vi "Bridge Null Offset.vi"(8 "error in (no error)":errorcluster, 11 "DAQmxAI in":refnum<class "DAQmxAI.lvclass">) -> (0 "error out":errorcluster, 3 "DAQmxAI out":refnum<class "DAQmxAI.lvclass">)   [LabVIEW 2023, in "VolatusDAQ.lvlib" / "DAQmxAI.lvclass"]
uses:
  DAQmxAI.lvclass
  DAQmxAI.lvclass/DAQmxAI.ctl
  Volatus/Module/Module.lvclass
  lv-vecto/Vecto/Group DBL/Group DBL.lvclass
  9ff7c66f-9138-48a5-beec-35436b15b101.vi
  C:/dev/volatus/mts-volatus-super/libs/lv-vecto/Vecto/Group/Group.lvclass
  C:/dev/volatus/mts-volatus-super/libs/lv-vecto/Vecto/Group DBL/Group DBL.lvclass
  C:/dev/volatus/mts-volatus-super/libs/lv-volatus/Volatus/Module/Module.lvclass
  C:/dev/volatus/mts-volatus-super/libs/lv-volatus/VolatusDAQ/DAQmxAI/DAQmxAI.lvclass
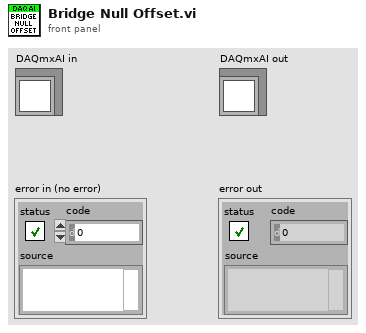
[diagram p1: front panel]
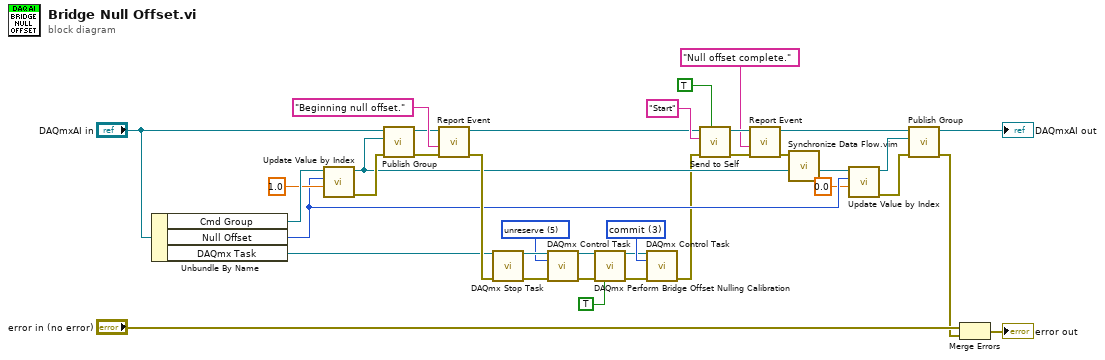
[diagram p0: block diagram]
diagram:
  w4 = 3 items=["verify"=2, "reserve"=4, "commit"=3, "unreserve"=5, "abort"=6] ("action")
  w7 = 5 items=["verify"=2, "reserve"=4, "commit"=3, "unreserve"=5, "abort"=6] ("action")
  n1 = Unbundle By Name("DAQmxAI in") -> ("Cmd Group"=w26:refnum<class "Group DBL.lvclass">, "Null Offset"=w21:i32, "DAQmx Task"=w35:refnum<k21>)
  n2 = call "Update Value by Index.vi"("Scaled"=1.0, "Index"=w21, "Group in"=w26) -> ("error out"=w23:errorcluster, "Group out"=w15:refnum<class "Group DBL.lvclass">)  [unwired: 7 in]
  n3 = call "Publish Group.vi"("error in (no error)"=w23, "Group"=w15, "Module in"="DAQmxAI in") -> ("error out"=w22:errorcluster, "Module out"=w24:refnum<class "DAQmxAI.lvclass">)  [unwired: 7 in]
  n4 = call "Report Event.vi"("error in (no error)"=w22, "Message"="Beginning null offset.", "Module in"=w24) -> ("error out"=w36:errorcluster, "Module out"=w30:refnum<class "DAQmxAI.lvclass">)  [unwired: 7 in]
  n5 = call <vilib>:"DAQmx Stop Task.vi"("task/channels in"=w35, "error in"=w36) -> ("task out"=w8:refnum<k21>, "error out"=w9:errorcluster)  [unwired: 12 in]
  n6 = call <vilib>:"DAQmx Control Task.vi"("task/channels in"=w8, "action"=w7, "error in"=w9) -> ("task out"=w6:refnum<k21>, "error out"=w5:errorcluster)  [unwired: 11 in]
  n7 = call <vilib>:"DAQmx Perform Bridge Offset Nulling Calibration.vi"("task/channels in"=w6, "error in"=w5, "skip unsupported channels"=TRUE) -> ("task out"=w3:refnum<k21>, "error out"=w2:errorcluster)  [unwired: 11 in]
  n8 = call <vilib>:"DAQmx Control Task.vi"("task/channels in"=w3, "action"=w4, "error in"=w2) -> ("error out"=w1:errorcluster)  [unwired: 11 in, 1 out]
  n9 = call "Send to Self.vi"("High Priority (F)"=TRUE, "error in (no error)"=w1, "Message ID"="Start", "Module in"=w30) -> ("error out"=w31:errorcluster, "Module out"=w28:refnum<class "DAQmxAI.lvclass">)  [unwired: 6 in]
  n10 = call "Report Event.vi"("error in (no error)"=w31, "Message"="Null offset complete.", "Module in"=w28) -> ("error out"=w16:errorcluster, "Module out"=w19:refnum<class "DAQmxAI.lvclass">)  [unwired: 7 in]
  n11 = call "Synchronize Data Flow.vim"("input 3"=w15, "input 1"=w16) -> ("output 3"=w14:refnum<class "Group DBL.lvclass">)  [unwired: 2 in, 3 out]
  n12 = call "Update Value by Index.vi"("Scaled"=0.0, "Index"=w21, "Group in"=w14) -> ("error out"=w17:errorcluster, "Group out"=w18:refnum<class "Group DBL.lvclass">)  [unwired: 7 in]
  n13 = call "Publish Group.vi"("error in (no error)"=w17, "Group"=w18, "Module in"=w19) -> ("error out"=w10:errorcluster, "Module out"=→"DAQmxAI out":refnum<class "DAQmxAI.lvclass">)  [unwired: 7 in]
  n14 = Merge Errors("error in (no error)", w10) -> (→"error out":errorcluster)
